vi "Add Waveforms from ListBox.vi"(5 "UI Refs":T2, 6 "error in (no error)":errorcluster, 7 "Wfm Ref LUT":variant, 8 "CD Settings in":T3 {"CD Task Dependency Ref" format="%.0x"; "CD Task Dependency" format="%.0x"}, 9 "Custom Device Ref in":T1 format="%.0x") -> (0 "error out":errorcluster, 1 "Wfm Ref LUT out":variant, 2 "CD Settings out":T3 {"CD Task Dependency Ref" format="%.0x"; "CD Task Dependency" format="%.0x"}, 3 "Custom Device Ref out":T1 format="%.0x")   [LabVIEW 2014, in "Waveform-Processing-Custom-Device System Explorer.lvlib"]
uses:
  Waveform-Processing-Custom-Device System Explorer.lvlib
  Shared/Custom Device Settings.ctl
  <vilib>/NI Veristand/Custom Device API/Custom Device Item Ref.ctl
  Types/UI Refs Ctl.ctl
  <vilib>/NI Veristand/Custom Device API/Custom Device Pointer.ctl
  NationalInstruments.VeriStand.SystemStorage
  <vilib>/NI Veristand/Custom Device API/Custom Device API.lvlib
  Shared/Waveform-Processing-Custom-Device Shared.lvlib
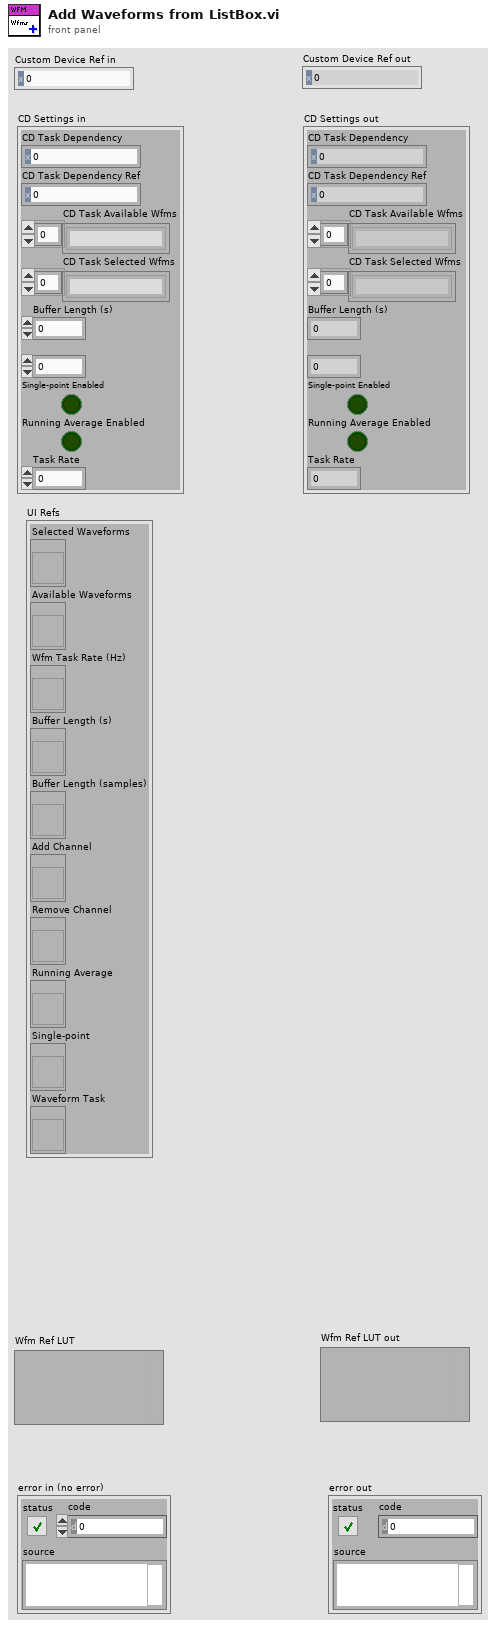
[diagram p1: front panel]
types:
  T1 = typedef "Custom Device API.lvlib/Custom Device Item Ref.ctl" = u64
  T2 = typedef "Waveform-Processing-Custom-Device Shared.lvlib/UI Refs Ctl.ctl" = cluster{"Selected Waveforms":refnum<vi>, "Available Waveforms":refnum<vi>, "Wfm Task Rate (Hz)":refnum<vi>, "Buffer Length (s)":refnum<vi>, "Buffer Length (samples)":refnum<vi>, "Add Channel":refnum<vi>, "Remove Channel":refnum<vi>, "Running Average":refnum<vi>, "Single-point":refnum<vi>, "Waveform Task":refnum<vi>}
  T3 = typedef "Waveform-Processing-Custom-Device Shared.lvlib/Custom Device Settings.ctl" = cluster{"CD Task Dependency":T1, "CD Task Dependency Ref":T1, "CD Task Available Wfms":string[], "CD Task Selected Wfms":string[], "Buffer Length (s)":dbl, "Buffer Length (samples)":u32, "Single-point Enabled":bool, "Running Average Enabled":bool, "Task Rate":dbl}
  T4 = typedef "Custom Device API.lvlib/Custom Device Pointer.ctl" = refnum<k24>
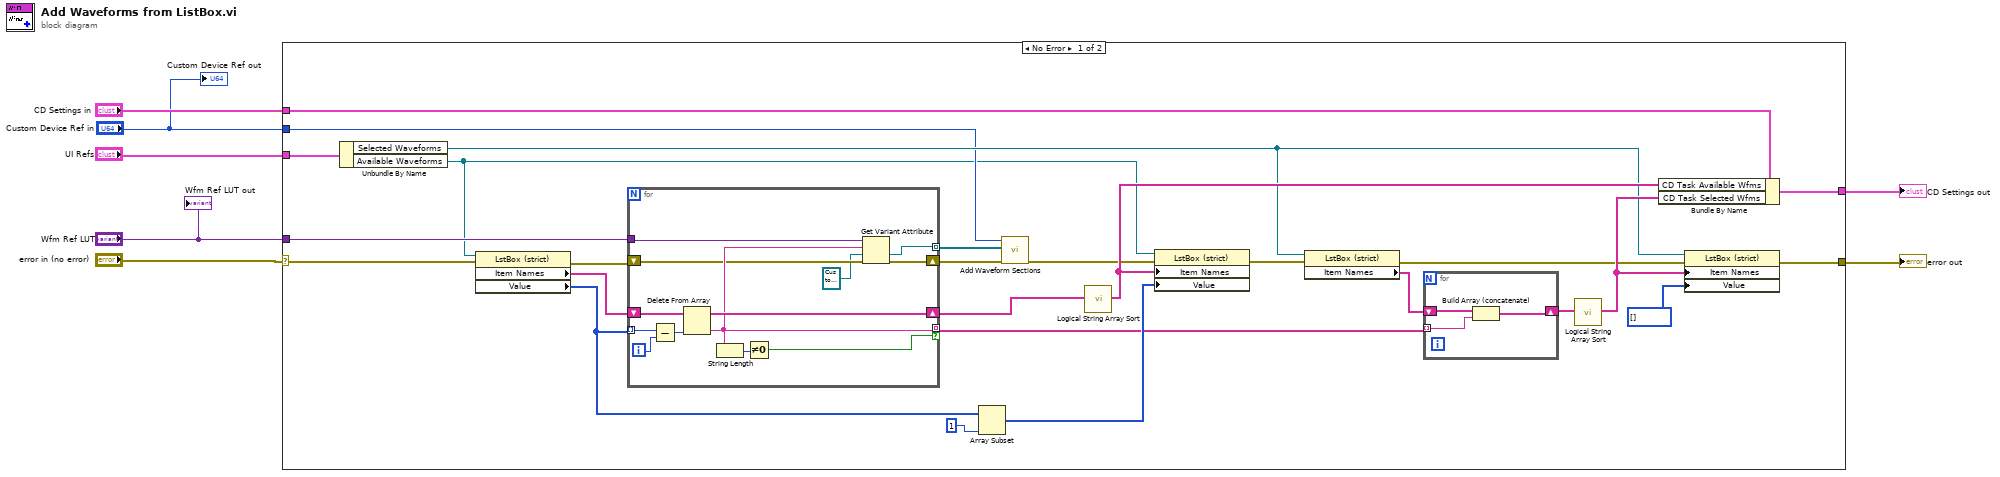
[diagram p0: block diagram]
diagram:
  n1 = case shown="No Error" "error in (no error)" {
    selector: "error in (no error)" -> [w13 w50]
    tunnel: [w26 w51] -> w7
    tunnel: "CD Settings in" -> [w25 w51]
    tunnel: [w8 w50] -> w5
    tunnel: "UI Refs" -> [w21 _]
    tunnel: "Wfm Ref LUT" -> [w18 _]
    tunnel: "Custom Device Ref in" -> [w15 _]
    frame No Error {
      n2 = Unbundle By Name(w21) -> ("Selected Waveforms"=w20:refnum<vi>, "Available Waveforms"=w12:refnum<vi>)
      n3 = property on="Property Node" class="LstBox (strict)"(reference=w12, error in=w13) -> (error out=w11:errorcluster, "Item Names"=w9:string[], "Value"=w10:i32[])  [unwired: 1 out]
      n4 = for {
        tunnel: w10 -> [w46] mode=indexing
        shift-right: [w48] -> w28
        shift-left: w9 -> [w49]
        tunnel: [w42] -> w23 mode=indexing if=w38
        tunnel: w18 -> [w43]
        shift-right: [w40] -> w17
        shift-left: w11 -> [w41]
        tunnel: [w39] -> w14 mode=indexing
        i -> [w47]
        n5 = Subtract(x=w46, y=w47) -> (x-y=w45:i32)
        n6 = Delete From Array(array=w49, index=w45) -> (deleted portion=w42:string, array with subset deleted=w48:string[])  [unwired: 1 in]
        n7 = String Length(string=w42) -> (length=w44:i32)
        n8 = Not Equal To 0?(x=w44) -> (x != 0?=w38:bool)
        n9 = Get Variant Attribute(Variant=w43, name=w42, default value (empty Variant)=T4 refnum ("Node Pointer"), error in=w41) -> (value=w39:T4, error out=w40:errorcluster)  [unwired: 2 out]
      }
      n10 = Array Subset(array=w10, length=1) -> (w32:i32[])  [unwired: 1 in]
      n11 = call "Add Waveform Sections.vi"("error in"=w17, "Wfm Pointers"=w14, "CustomDevice Ref"=w15) -> ("error out"=w16:errorcluster)  [unwired: 7 in, 1 out]
      n12 = call "Logical String Array Sort.vi"("Unsorted List"=w28) -> ("Sorted List"=w29:string[])  [unwired: 18 in]
      n13 = property on="Property Node" class="LstBox (strict)"(reference=w12, error in=w16, "Item Names"=w29, "Value"=w32) -> (error out=w22:errorcluster)  [unwired: 1 out]
      n14 = property on="Property Node" class="LstBox (strict)"(reference=w20, error in=w22) -> (error out=w24:errorcluster, "Item Names"=w27:string[])  [unwired: 1 out]
      n15 = for {
        tunnel: w23 -> [w35] mode=indexing
        shift-right: [w34] -> w30
        shift-left: w27 -> [w36]
        n16 = Build Array (concatenate)(w36, w35) -> (w34:string[])
      }
      n17 = call "Logical String Array Sort.vi"("Unsorted List"=w30) -> ("Sorted List"=w31:string[])  [unwired: 18 in]
      n18 = Bundle By Name(cluster=w25, "CD Task Available Wfms"=w29, "CD Task Selected Wfms"=w31) -> (w26:T3)
      n19 = property on="Property Node" class="LstBox (strict)"(reference=w20, error in=w24, "Item Names"=w31, "Value"=i32[] [] ("Waveforms to Process")) -> (error out=w8:errorcluster)  [unwired: 1 out]
    }
    frame Error {
    }
  }
  "CD Settings out" <- w7
  "error out" <- w5
  "Custom Device Ref out" <- "Custom Device Ref in"
  "Wfm Ref LUT out" <- "Wfm Ref LUT"
